vi "Baseline Header To Tags.vi"(2 "error in":errorcluster, 3 "IFD Baseline":T3={"NewSubFileType"=2, "ImageWidth"=1112, "ImageHeight"=3152, "BitsPerSample"=64, "Compression"=1, "PhotometricInterpretation"=1, "StripOffsets"=[8], "SamplesPerPixel"=1, "RowsPerStrip"=3152, "StripByteCounts"=[], "ResolutionUnit"=1, "SampleFormat"=3} {"SampleFormat" items=["UINT"=1, "INT"=2, "FP"=3, "VOID"=4, "COMPLEXINT"=5, "COMPLEXFP"=6]; "NewSubFileType" items=["FILETYPE_REDUCEDIMAGE"=1, "FILETYPE_PAGE"=2, "FILETYPE_MASK"=4]; "Compression" items=["COMPRESSION_NONE"=1, "COMPRESSION_CCITTRLE"=2, "COMPRESSION_CCITTFAX3"=3, "COMPRESSION_CCITTFAX4"=4, "COMPRESSION_LZW"=5, "COMPRESSION_OJPEG"=6, "COMPRESSION_JPEG"=7, "COMPRESSION_NEXT"=32766, "COMPRESSION_CCITTRLEW"=32771, "COMPRESSION_PACKBITS"=32773, "COMPRESSION_THUNDERSCAN"=32809, "COMPRESSION_IT8CTPAD"=32895, "COMPRESSION_IT8LW"=32896, "COMPRESSION_IT8MP"=32897, "COMPRESSION_IT8BL"=32898, "COMPRESSION_PIXARFILM"=32908, "COMPRESSION_PIXARLOG"=32909, "COMPRESSION_DEFLATE"=32946, "COMPRESSION_ADOBE_DEFLATE"=8, "COMPRESSION_DSC"=32947, "COMPRESSION_JBIG"=34661, "COMPRESSION_SGILOG"=34676, "COMPRESSION_SGILOG24"=34677, "COMPRESSION_JP2000"=34712]; "PhotometricInterpretation" items=["PHOTOMETRIC_MINISWHITE"=0, "PHOTOMETRIC_MINISBLACK"=1, "PHOTOMETRIC_RGB"=2, "PHOTOMETRIC_PALETTE"=3, "PHOTOMETRIC_MASK"=4, "PHOTOMETRIC_SEPARATED"=5, "PHOTOMETRIC_YCBCR"=6, "PHOTOMETRIC_CIELAB"=8, "PHOTOMETRIC_ICCLAB"=9, "PHOTOMETRIC_ITULAB"=10, "PHOTOMETRIC_LOGL"=32844, "PHOTOMETRIC_LOGLUV"=32845, "CFA"=32803, "LinearRaw"=34892, "DEPTH"=51177]; "ResolutionUnit" items=["RESUNIT_NONE"=1, "RESUNIT_INCH"=2, "RESUNIT_CENTIMETER"=3]}) -> (0 "error out":errorcluster, 1 "Tags":T2(array[cluster]))   [LabVIEW 2020, in "LV Tiff.lvlib"]
uses:
  LV Tiff.lvlib
  Baseline Tags 1.ctl
  <vilib>/Utility/Data Type/Type Definitions/Data Type.ctl
  <vilib>/Utility/Data Type/NI_Data Type.lvlib
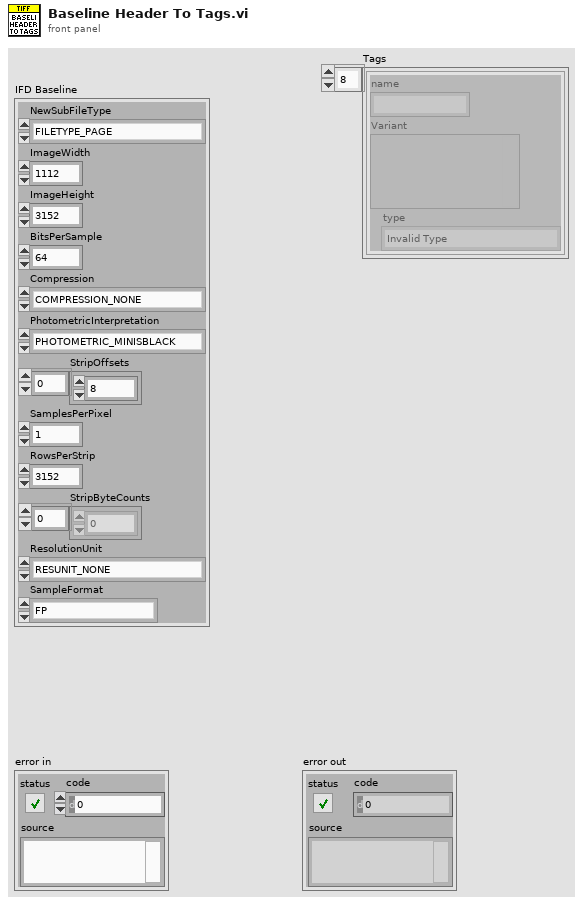
[diagram p1: front panel]
types:
  T1 = typedef "NI_Data Type.lvlib/Data Type.ctl" = enum8{"Invalid Type", "Void", "I8", "I16", "I32", "I64", "U8", "U16", "U32", "U64", "Single Float", "Double Float", "Extended Float", "Single Complex", "Double Complex", "Extended Complex", "Enum U8", "Enum U16", "Enum U32", "Enum U64", "Single Float With Unit", "Double Float With Unit", "Extended Float With Unit", "Single Complex with Unit", "Double Complex with Unit", "Extended Complex with Unit", "Boolean", "String", "Path", "Picture", "Tag", "Array", "Cluster", "Variant", "LV Variant", "Waveform", "Timestamp", "Digital Waveform", "Digital Data", "ExpressData", "Refnum", "External Data", "VI", "Poly VI", "LabVIEW Class Instance", "Fixed Point", "Set Collection", "Map Collection"}
  T2 = cluster{"name":string, "Variant":variant, "type":T1}[]
  T3 = typedef "LV Tiff.lvlib/Baseline Tags 1.ctl" = cluster{"NewSubFileType":u32, "ImageWidth":u32, "ImageHeight":u32, "BitsPerSample":u16, "Compression":u16, "PhotometricInterpretation":u16, "StripOffsets":u32[], "SamplesPerPixel":u16, "RowsPerStrip":u32, "StripByteCounts":u32[], "ResolutionUnit":u16, "SampleFormat":u16}
  T4 = cluster{"name":string, "Variant":variant, "type":T1}
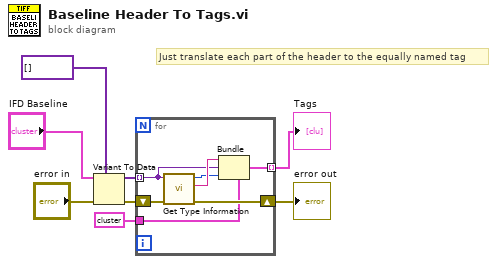
[diagram p0: block diagram]
diagram:
  # "Just translate each part of the header to the equally named tag"
  n1 = Variant To Data(error in="error in", type=variant[] [], Variant="IFD Baseline") -> (data=w7:variant[], error out=w6:errorcluster)
  n2 = for {
    tunnel: w7 -> [w14] mode=indexing
    tunnel: [w13] -> w3 mode=indexing
    shift-right: [w11] -> w4
    shift-left: w6 -> [w12]
    tunnel: T4 {"name"="", "Variant"=variant, "type"=enum."Invalid Type"} ("cluster") -> [w9]
    n3 = call <vilib>:"Get Type Information.vi"("error in (no error)"=w12, "variant"=w14) -> ("error out"=w11:errorcluster, "name"=w15:string, "type"=w10:T1)  [unwired: 5 in, 2 out]
    n4 = Bundle(cluster=w9, "name"=w15, "Variant"=w14, "type"=w10) -> (w13:T4)
  }
  "error out" <- w4
  "Tags" <- w3
